vi "Test_LogLevelFilter_FilterSetInfo_OnlyInfoLogged.vi"(8 "error in (no error)":errorcluster, 11 "TestCase in":refnum<class "TestLogFilter.lvclass">) -> (0 "error out":errorcluster, 3 "TestCase out":refnum<class "TestLogFilter.lvclass">)   [LabVIEW 2019, in "TestLogFilter.lvclass"]
uses:
  TestLogFilter.lvclass
  Source/Composed Log/Types/Log Level.ctl
  Source/Composed Log/LoggerReference/LoggerReference.lvclass/LoggerReference.ctl
  Source/LVQueue Sink/LVQueue Sink.lvclass/LVQueue Sink.ctl
  26d7161e-c156-4889-977f-6ef5c4e245d6.vi
  Source/Composed Log/LoggerReference/Return Aggregate Queues.vi
  Source/Composed Log/LoggerReference/Add Aggregate Log.vi
  26d7161e-c156-4889-977f-6ef5c4e245d6.vi/f3741cfb-6292-4ed9-af24-82bf0df9f24a.vi
  Source/Composed Log/LoggerReference/Log.vi
  Source/Composed Log/LoggerReference/Get Valid Event Time.vi
  Source/Composed Log/LoggerReference/Send Add Sink.vi
  Source/Composed Log/LoggerReference/Remove Stale Logs.vi
  Source/Filters/Event Level Filter/Event Level Filter.lvclass
  C:/CS/Log/Source/Composed Log/ILogFilter/ILogFilter.lvclass
  Source/LVQueue Sink/LVQueue Sink.lvclass
  C:/CS/Log/Source/Composed Log/Log Sink/Log Sink.lvclass
  Source/Composed Log/Application Logger/Launch Worker Loop.vi
  Source/Composed Log/LoggerReference/Initialize Logger Instance.vi
  Source/Composed Log/LoggerReference/LoggerReference.lvclass
  Source/Composed Log/IErrorFormat/IErrorFormat.lvclass
  Source/Composed Log/Log Sink/Log Sink.lvclass
  <vilib>/addons/_JKI Toolkits/VI Tester/TestCase.llb/TestCase.lvclass
  Source/Composed Log/Composed Log.lvlib
  C:/Program Files (x86)/National Instruments/LabVIEW 2019/vi.lib/addons/_JKI Toolkits/VI Tester/TestCase.llb/TestCase.lvclass
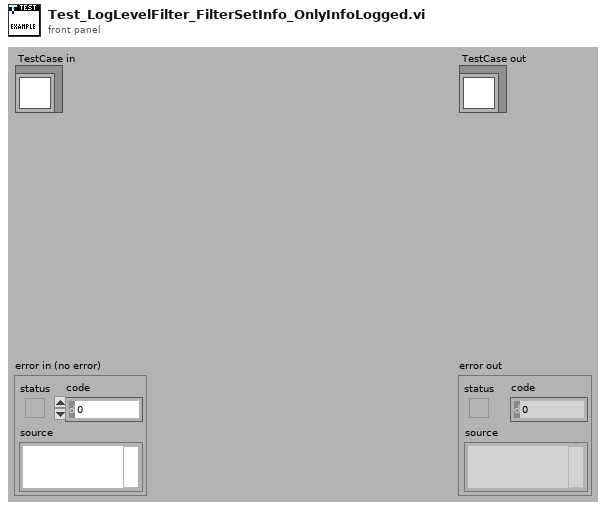
[diagram p1: front panel]
types:
  T1 = typedef "Composed Log.lvlib/Log Level.ctl" = enum16{"Debug", "Info", "Warning", "Error", "Critical"}
  T2 = cluster{"Debug":bool, "Info":bool, "Warning":bool, "Error":bool, "Critical":bool}
  T3 = typedef "Composed Log.lvlib/Log Packet.ctl" = cluster{"Data To Log":string, "Source":string, "Event Level":T1, "Event Time":timestamp}
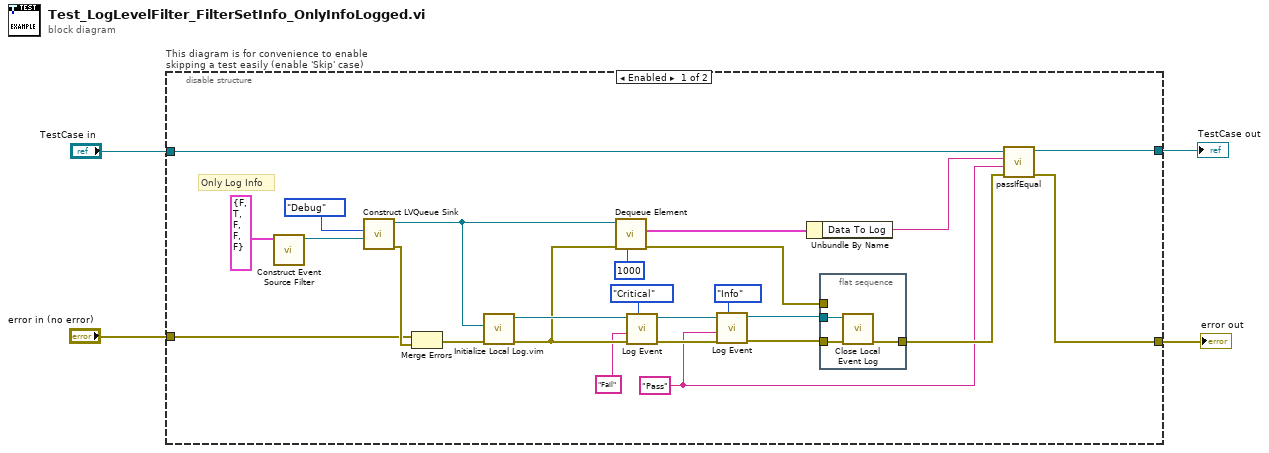
[diagram p0: block diagram]
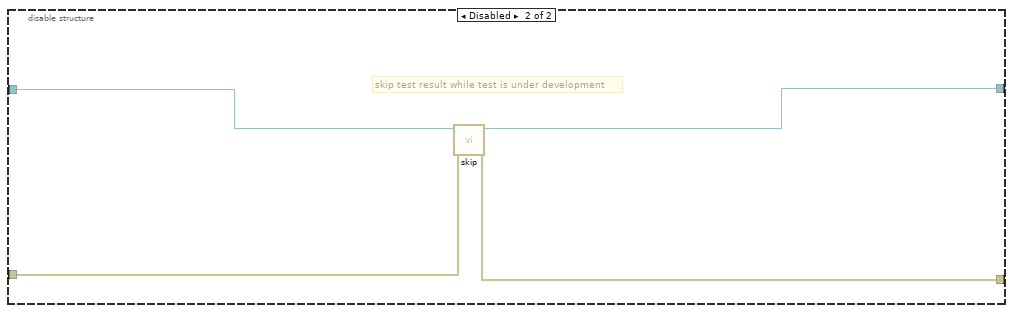
[diagram p2: hidden frame]
diagram:
  n1 = disable-structure "This diagram is for convenience to enable skipping a test easily (enable 'Skip' case)" shown="Enabled" {
    disable-tunnel: "TestCase in" -> [w21 w36]
    disable-tunnel: [w20 w34] -> w1
    disable-tunnel: [w19 w35] -> w3
    disable-tunnel: "error in (no error)" -> [w18 w33]
    frame Enabled {
      w6 = "Pass" ("Data To Log")
      # "Only Log Info"
      n2 = call "Construct Event Source Filter.vi"("Levels to Include (All)"=T2 {"Debug"=FALSE, "Info"=TRUE, "Warning"=FALSE, "Error"=FALSE, "Critical"=FALSE}) -> ("Event Level Filter out"=w14:refnum<class "Event Level Filter.lvclass">)  [unwired: 10 in]
      n3 = call "Construct LVQueue Sink.vi"("Log Filter"=w14, "LogLevel"=Log_Level."Debug") -> ("error out"=w26:errorcluster, "LVQueue Sink out"=w24:refnum<class "LVQueue Sink.lvclass">)  [unwired: 8 in]
      n4 = Merge Errors(w18, w26) -> (w25:errorcluster)
      n5 = call "Initialize Local Log.vim"("error in (no error)"=w25, "Startup Sink(s)"=w24) -> ("error out"=w16:errorcluster, "Log Instance Reference"=w17:refnum<class "LoggerReference.lvclass">)  [unwired: 7 in, 1 out]
      n6 = call "Dequeue Element.vi"("timeout in ms (-1)"=1000, "error in (no error)"=w16, "LVQueue Sink in"=w24) -> ("error out"=w29:errorcluster, "Log Packet"=w27:T3)  [unwired: 5 in, 2 out]
      n7 = call "Log Event.vi"("Event Level"=Log_Level."Critical", "error in (no error)"=w16, "Data To Log"="Fail", "Log Instance"=w17) -> ("error out"=w12:errorcluster, "Log Instance Out"=w13:refnum<class "LoggerReference.lvclass">)  [unwired: 6 in]
      n8 = call "Log Event.vi"("Event Level"=Log_Level."Info", "error in (no error)"=w12, "Data To Log"=w6, "Log Instance"=w13) -> ("error out"=w10:errorcluster, "Log Instance Out"=w11:refnum<class "LoggerReference.lvclass">)  [unwired: 6 in]
      n9 = Unbundle By Name(w27) -> ("Data To Log"=w23:string)
      n10 = flat-sequence {
        tunnel: [w31] -> w28
        tunnel: w10 -> [w32]
        tunnel: w29 -> [_]
        tunnel: w11 -> [w30]
        frame #0 {
          n11 = call "Close Local Event Log.vi"("error in (no error)"=w32, "Log Instance"=w30) -> ("error out"=w31:errorcluster)  [unwired: 9 in]
        }
      }
      n12 = call-dynamic "passIfEqual.vi"("error in (no error)"=w28, "y"=w6, "x"=w23, "TestCase in"=w21) -> ("error out"=w19:errorcluster, "TestCase out"=w20:refnum<class "TestLogFilter.lvclass">)  [unwired: 6 in]
    }
    frame Disabled {
      # "skip test result while test is under development"
      n13 = call <vilib>:"skip.vi"("error in (no error)"=w33, "TestCase in"=w36) -> ("error out"=w35:errorcluster, "TestCase out"=w34:refnum<class "TestLogFilter.lvclass">)  [unwired: 8 in]
    }
  }
  "error out" <- w3
  "TestCase out" <- w1
